vi "Check message.vi"(8 "error in (no error)":errorcluster, 9 "isAcommand":bool, 10 "message in":string) -> (0 "error out":errorcluster, 1 "valid":bool, 2 "message":string, 4 "not empty":bool)   [LabVIEW 2018]
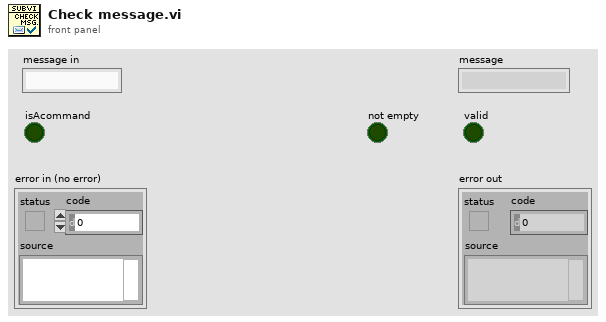
[diagram p1: front panel]
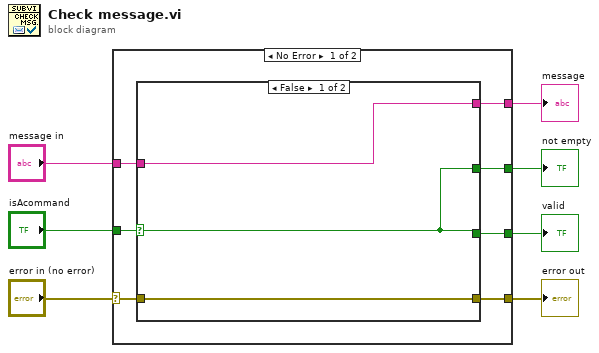
[diagram p0: block diagram]
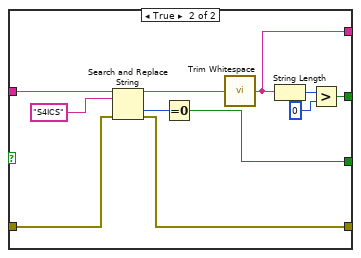
[diagram p2: hidden frame]
diagram:
  n1 = case shown="No Error" "error in (no error)" {
    selector: "error in (no error)" -> [w13 w29]
    tunnel: "message in" -> [w14 _]
    tunnel: [w12 w29] -> w5
    tunnel: [w9 _] -> w2
    tunnel: [w10 _] -> w3
    tunnel: [w11 _] -> w4
    tunnel: "isAcommand" -> [w8 _]
    frame No Error {
      n2 = case shown="False" w8 {
        selector: w8 -> [w16 _]
        tunnel: w14 -> [w17 w26]
        tunnel: w13 -> [w15 w23]
        tunnel: [w15 w22] -> w12
        tunnel: [w17 w20] -> w11
        tunnel: [w16 w19] -> w10
        tunnel: [w16 w18] -> w9
        frame False {
        }
        frame True {
          n3 = Search and Replace String(input string=w26, search string="S4ICS", error in=w23) -> (result string=w21:string, offset past replacement=w24:i32, error out=w22:errorcluster)  [unwired: 5 in, 1 out]
          n4 = Equal To 0?(x=w24) -> (x = 0?=w18:bool)
          n5 = call <vilib>:"Trim Whitespace.vi"("string"=w21) -> ("trimmed string"=w20:string)  [unwired: 1 in]
          n6 = String Length(string=w20) -> (length=w27:i32)
          n7 = Greater?(x=w27, y=0) -> (0:w19:bool)
        }
      }
    }
    frame Error {
    }
  }
  "error out" <- w5
  "message" <- w4
  "not empty" <- w3
  "valid" <- w2
